vi "L0_ASIC_COMPLETE_TEST.vi"() -> ()   [LabVIEW 2009]
uses:
  <vilib>/Utility/NIReport.llb/NI_report.lvclass
  <vilib>/Utility/NIReport.llb/HTML/NI_HTML.lvclass
panel:
  out "Instrument VISA out":T1={"AWG VISA"="generadorpulsos", "Oscilloscope  VISA "="Oscilloscope", "Integration Board IP"="172.16.7.43", "connection ID"=refnum, "report out"=refnum, "report file path"=path "C:/Documents and Settings/CTA_LAB01/Desktop/L0_Asic/L0 Asic Test Data"}
  in  "Instrument VISA in":T1={"AWG VISA"="generadorpulsos", "Oscilloscope  VISA "="Oscilloscope", "Integration Board IP"="172.16.7.43", "connection ID"=refnum, "report out"=refnum, "report file path"=path "C:/Documents and Settings/CTA_LAB01/Desktop/L0_Asic/L0 Asic Test Data"}
  out "error out":errorcluster
  in  "error in":errorcluster
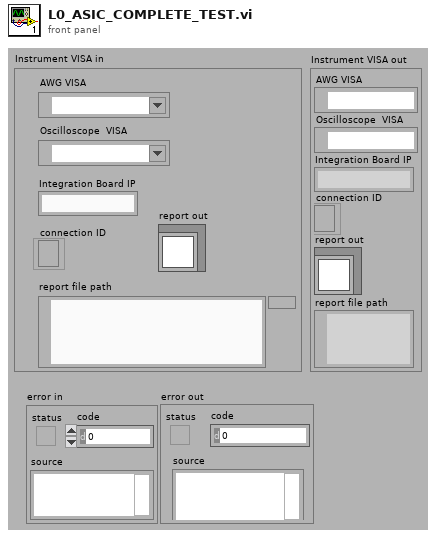
[diagram p1: front panel]
types:
  T1 = cluster{"AWG VISA":refnum<visa-resource-name>, "Oscilloscope  VISA ":refnum<visa-resource-name>, "Integration Board IP":string, "connection ID":refnum<k5>, "report out":refnum<class "NI_report.lvclass">, "report file path":path}
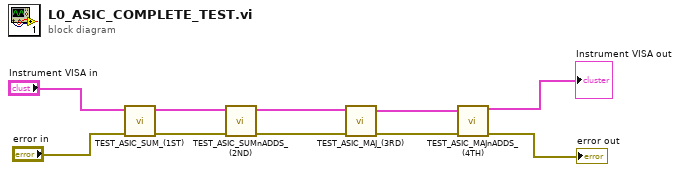
[diagram p0: block diagram]
diagram:
  n1 = call "TEST_ASIC_SUM_(1ST).vi"("error in"="error in", "Instrument VISA in"="Instrument VISA in") -> ("error out"=w4:errorcluster, "Instrument VISA out"=w9:T1)  [unwired: 8 in]
  n2 = call "TEST_ASIC_SUMnADDS_(2ND).vi"("Instrument VISA in"=w9, "error in"=w4) -> ("Instrument VISA out"=w6:T1, "error out"=w2:errorcluster)  [unwired: 12 in]
  n3 = call "TEST_ASIC_MAJ_(3RD).vi"("error in"=w2, "Instrument VISA in"=w6) -> ("error out"=w1:errorcluster, "Instrument VISA out"=w7:T1)  [unwired: 7 in, 1 out]
  n4 = call "TEST_ASIC_MAJnADDS_(4TH).vi"("Instrument VISA in"=w7, "error in"=w1) -> ("Instrument VISA out"=→"Instrument VISA out":T1, "error out"=→"error out":errorcluster)  [unwired: 12 in]
